vi "Get Calibration Sign (uSMC).vi"(4 "SM index":i32) -> (1 "Calibration Sign":bool)   [LabVIEW 2010, in "SignalWriterMH110203USBStepperMotor.lvclass"]
uses:
  SignalWriterMH110203USBStepperMotor.lvclass
  class_data.vi
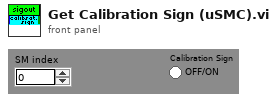
[diagram p1: front panel]
types:
  T1 = typedef "SignalWriterMH110203USBStepperMotor.lvclass/GoTo Control (uSMC).ctl" = cluster{"Step motor ID":string, "SMname":string, "Backlash":u16, "wait for input sygnal to start":bool, "use slow start/stop":bool, "units name":string, "Maximum speed":dbl, "speed":dbl, "step":u8, "point 1 ticks":i32, "point 2 ticks":i32, "point 1 units":dbl, "point 2 units":dbl, "Limit Switch standoff":dbl, "Zero Value":dbl, "Destination Position":dbl, "force backlash":bool, "power off when stop":bool, "POff delay":dbl, "positioner name":string, "R, Ohm":dbl, "I, mA":dbl, "Positioner's Type":u16, "Reset Direction":bool, "Manufacturer":string, "Model":string, "Scheme":string, "FirmwareVer":string}
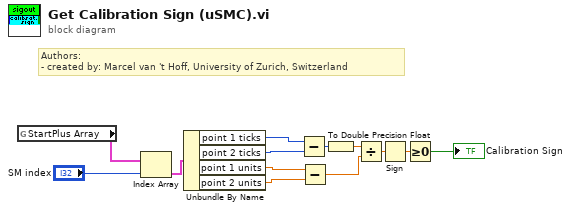
[diagram p0: block diagram]
diagram:
  # "Authors: \n- created by: Marcel van 't Hoff, University of Zurich, Switzerland"
  n1 = global read "class_data.vi" "StartPlus Array"() -> (w7:T1[])
  n2 = Index Array(array=w7, index="SM index") -> (element=w6:T1)
  n3 = Unbundle By Name(w6) -> ("point 1 ticks"=w5:i32, "point 2 ticks"=w4:i32, "point 1 units"=w3:dbl, "point 2 units"=w2:dbl)
  n4 = Subtract(x=w5, y=w4) -> (x-y=w8:i32)
  n5 = Subtract(x=w3, y=w2) -> (x-y=w9:dbl)
  n6 = To Double Precision Float(number=w8) -> (double precision float=w11:dbl)
  n7 = Divide(x=w11, y=w9) -> (x/y=w10:dbl)
  n8 = Sign(1:w10) -> (0:w12:dbl)
  n9 = Greater Or Equal To 0?(x=w12) -> (x >= 0?=→"Calibration Sign":bool)
